vi "AlliGator Enter User-defined Phasor Dialog.vi"(8 "Error In":errorcluster, 9 "Phasor Frequency":dbl[unit], 11 "Phasor Plot Name":string) -> (0 "Error Out":errorcluster, 1 "Cancelled?":bool, 3 "New Phasor (g, s)":T4, 4 "Message":string)   [LabVIEW 2021, in "AlliGator Phasor Graph.lvlib"]
doc: "User-entered phasor dialog."
uses:
  AlliGator Phasor Graph.lvlib
  Phasor/Phasor (g, s).ctl
  Phasor/Phasor (m, phi).ctl
  Phasor/Phasor.lvlib
panel:
  in  "Prefactor Type":enum32{"Exp. Amplitude", "Intensity Fraction"}(radio)
  in  "Cancel":bool
  in  "OK":bool
  in  "Double-Exponential":T1
  in  "Single-Lifetime":dbl[unit]
  out "User Message":string
  in  "Type of Phasor Definition":T2(radio)
  in  "Phasor (m, phi)":T3
  in  "Phasor (g, s)":T4
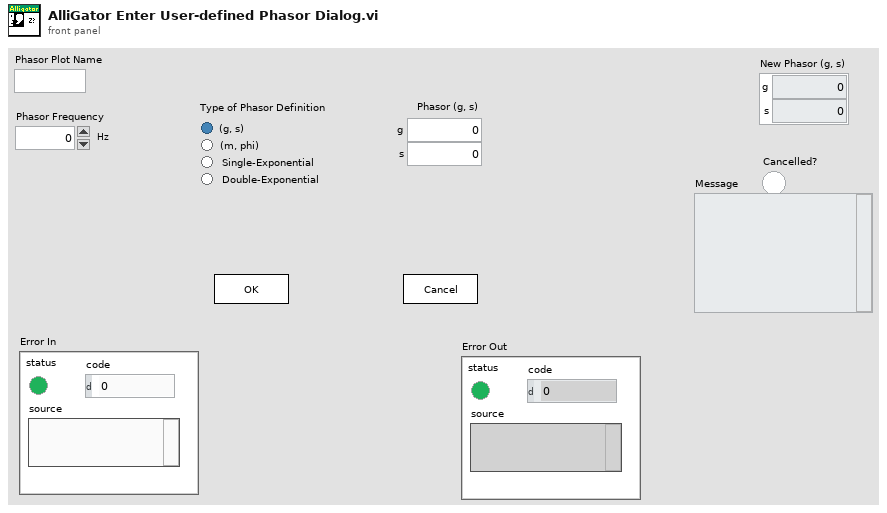
[diagram p1: front panel]
types:
  T1 = cluster{"Lifetime 1":dbl[unit], "Prefactor 1":dbl, "Lifetime 2":dbl[unit], "Prefactor 2":dbl}
  T2 = enum32{"(g, s)", "(m, phi)", "Single-Exponential", "Double-Exponential"}
  T3 = typedef "Phasor.lvlib/Phasor (m, phi).ctl" = cluster{"m":dbl, "phi":dbl}
  T4 = typedef "Phasor.lvlib/Phasor (g, s).ctl" = cluster{"g":dbl, "s":dbl}
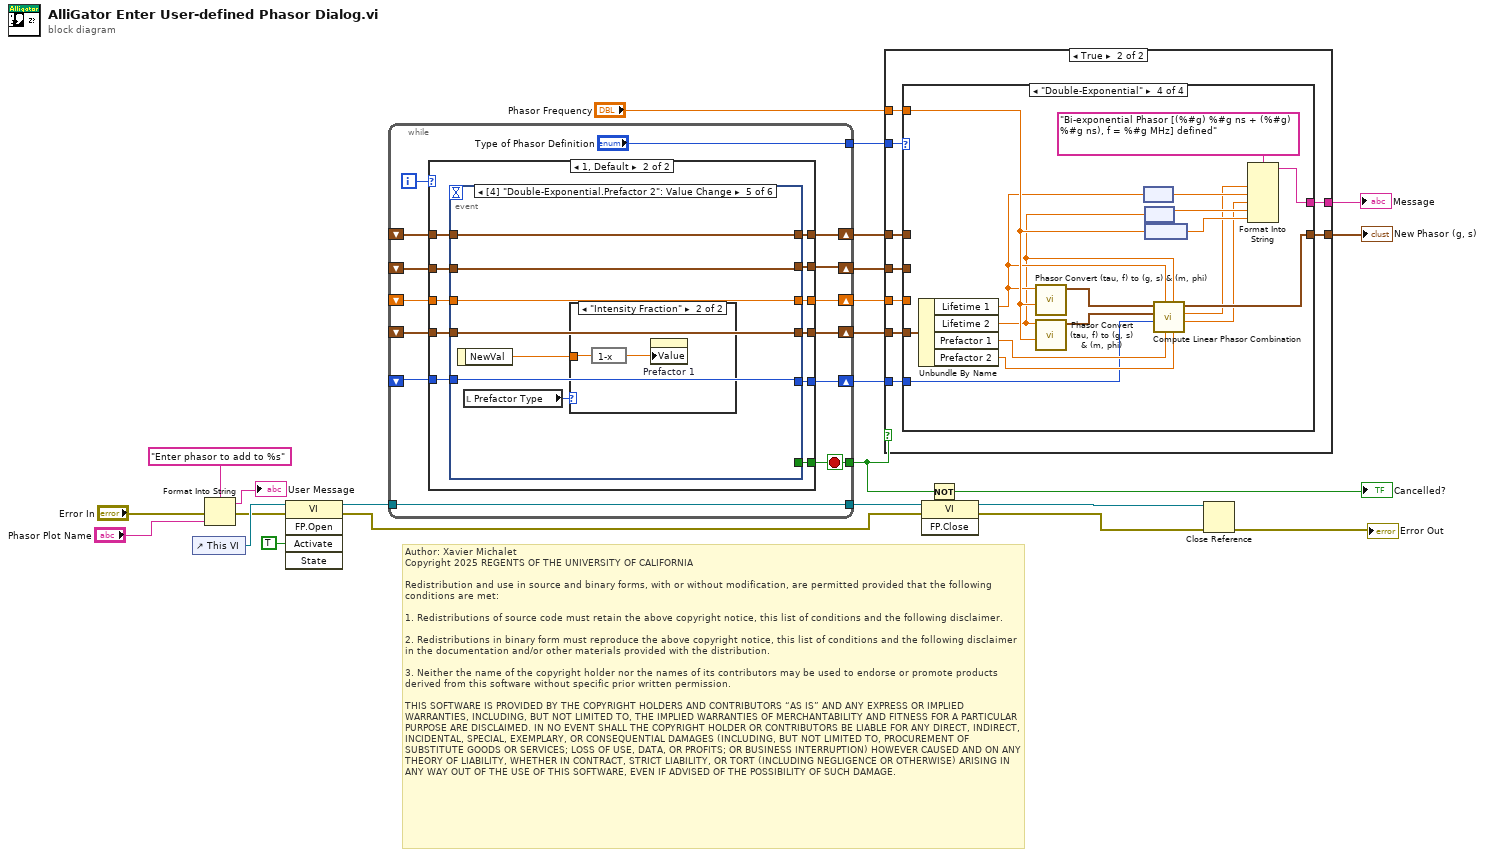
[diagram p0: block diagram]
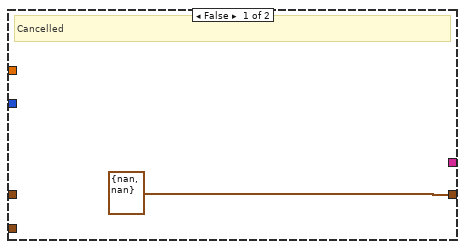
[diagram p2: hidden frame]
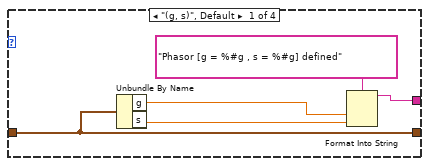
[diagram p3: hidden frame]
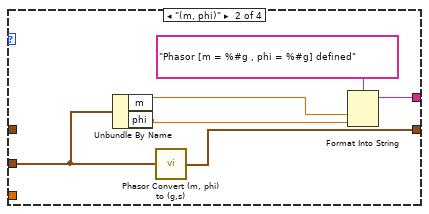
[diagram p4: hidden frame]
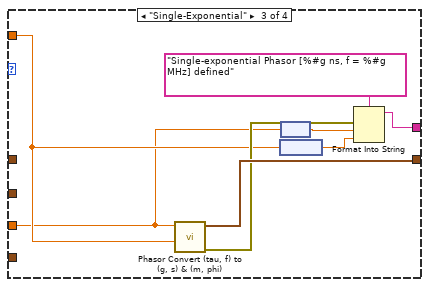
[diagram p5: hidden frame]
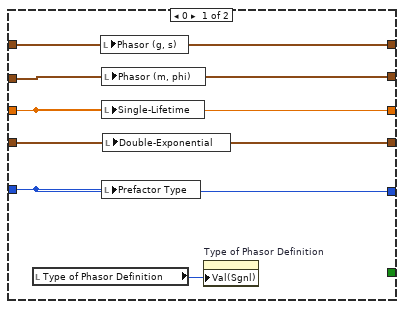
[diagram p6: hidden frame]
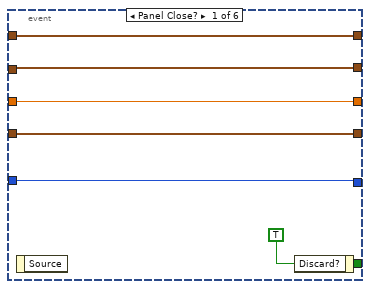
[diagram p7: hidden frame]
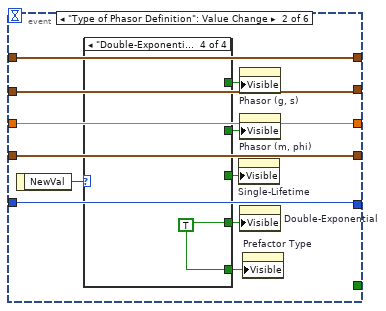
[diagram p8: hidden frame]
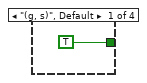
[diagram p9: hidden frame]
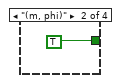
[diagram p10: hidden frame]
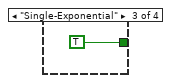
[diagram p11: hidden frame]
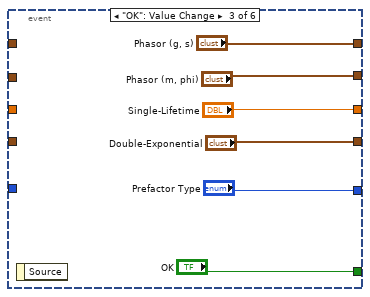
[diagram p12: hidden frame]
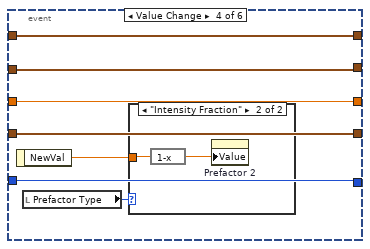
[diagram p13: hidden frame]
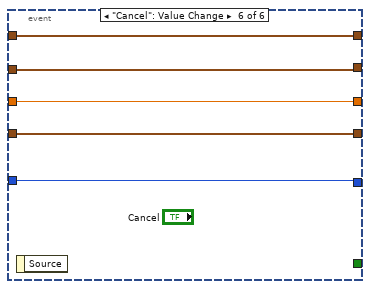
[diagram p16: hidden frame]
diagram:
  # "Author: Xavier Michalet\nCopyright 2025 REGENTS OF THE UNIVERSITY OF CALIFORNIA\n\nRedistribution and use in source and binary forms, with or without modification, are permitted provided that the following conditions are met:\n\n1. Redistributions of source code must retain the above copyright notice, this list of conditions and the following disclaimer.\n\n2. Redistributions in binary form must reproduce the above copyright notice, this list of conditions and the following disclaimer in the documentation and/or other materials provided with the distribution.\n\n3. Neither the name of the copyright holder nor the names of its contributors may be used to endorse or promote products derived from this software without specific prior written permission.\n\nTHIS SOFTWARE IS PROVIDED BY THE COPYRIGHT HOLDERS AND CONTRIBUTORS “AS IS” AND ANY EXPRESS OR IMPLIED WARRANTIES, INCLUDING, BUT NOT LIMITED TO, THE IMPLIED WARRANTIES OF MERCHANTABILITY AND FITNESS FOR A PARTICULAR PURPOSE ARE DISCLAIMED. IN NO EVENT SHALL THE COPYRIGHT HOLDER OR CONTRIBUTORS BE LIABLE FOR ANY DIRECT, INDIRECT, INCIDENTAL, SPECIAL, EXEMPLARY, OR CONSEQUENTIAL DAMAGES (INCLUDING, BUT NOT LIMITED TO, PROCUREMENT OF SUBSTITUTE GOODS OR SERVICES; LOSS OF USE, DATA, OR PROFITS; OR BUSINESS INTERRUPTION) HOWEVER CAUSED AND ON ANY THEORY OF LIABILITY, WHETHER IN CONTRACT, STRICT LIABILITY, OR TORT (INCLUDING NEGLIGENCE OR OTHERWISE) ARISING IN ANY WAY OUT OF THE USE OF THIS SOFTWARE, EVEN IF ADVISED OF THE POSSIBILITY OF SUCH DAMAGE."
  n1 = control-ref of="This VI"() -> (w24:refnum<vi>)
  n2 = Format Into String(format string="Enter phasor to add to %s", error in="Error In", "Phasor Plot Name") -> (resulting string=→"User Message":string, error out=w13:errorcluster)  [unwired: 1 in]
  n3 = invoke class="VI" method="FP.Open"(reference=w24, error in=w13, "Activate"=TRUE ("Activate?")) -> (reference out=w22:refnum<vi>, error out=w18:errorcluster)  [unwired: 2 in, 3 out]
  n4 = while {
    shift-right: [w33] -> w8
    shift-left: _ -> [w37]
    shift-right: [w32] -> w6
    shift-left: _ -> [w36]
    shift-right: [w31] -> w4
    shift-left: _ -> [w35]
    shift-right: [w30] -> w3
    shift-left: _ -> [w34]
    tunnel: ["Type of Phasor Definition"] -> w14
    tunnel: [w28] -> w15
    tunnel: w22 -> [w27]
    tunnel: [w27] -> w21
    shift-right: [w25] -> w1
    shift-left: _ -> [w26]
    i -> [w38]
    stop <- w28 stop-if-true
    n5 = case shown="1, Default" w38 {
      tunnel: [_ w55] -> w28
      tunnel: w37 -> [w44 w54]
      tunnel: w36 -> [w43 w52]
      tunnel: w35 -> [w42 w50]
      tunnel: w34 -> [w41 w48]
      tunnel: [w44 w53] -> w33
      tunnel: [w43 w51] -> w32
      tunnel: [w42 w49] -> w31
      tunnel: [w41 w47] -> w30
      tunnel: w26 -> [w39 w45]
      tunnel: [w39 w46] -> w25
      frame 0 {
        n6 = local read "Type of Phasor Definition"() -> (w40:T2)
        n7 = local write "Phasor (g, s)"(w44) -> ()
        n8 = local write "Phasor (m, phi)"(w43) -> ()
        n9 = local write "Single-Lifetime"(w42) -> ()
        n10 = local write "Prefactor Type"(w39) -> ()
        n11 = local write "Double-Exponential"(w41) -> ()
        n12 = property on="Type of Phasor Definition" class="RadioBtnsControl (strict)"("Val(Sgnl)"=w40) -> ()  [unwired: 2 in, 2 out]
      }
      frame 1, Default {
        n13 = event shown="[4] \"Double-Exponential.Prefactor 2\": Value Change" {
          selector: _ -> [_ _ _ _ _ _]
          dyn-events: _ -> [_ _ _ _ _ _]
          timeout: _ -> [_ _ _ _ _ _]
          tunnel: [w61 _ "OK" _ _ _] -> w55
          tunnel: w54 -> [w60 w67 _ w89 w98 w105]
          tunnel: [w60 w67 "Phasor (g, s)" w89 w98 w105] -> w53
          tunnel: w52 -> [w59 w66 _ w88 w97 w104]
          tunnel: [w59 w66 "Phasor (m, phi)" w88 w97 w104] -> w51
          tunnel: w50 -> [w58 w65 _ w87 w96 w103]
          tunnel: [w58 w65 "Single-Lifetime" w87 w96 w103] -> w49
          tunnel: w48 -> [w57 w64 _ w86 w95 w102]
          tunnel: [w57 w64 "Double-Exponential" w86 w95 w102] -> w47
          tunnel: [w56 w63 "Prefactor Type" w85 w94 w101] -> w46
          tunnel: w45 -> [w56 w63 _ w85 w94 w101]
          event Panel Close? {
            w61 = TRUE ("Discard?")
            n14 = event-data() -> ()  [unwired: 1 in, 1 out]
            n15 = event-data("Discard?"=w61) -> ()  [unwired: 1 in, 1 out]
          }
          event "Type of Phasor Definition": Value Change {
            n16 = event-data() -> ("NewVal"=w72:T2)  [unwired: 1 in]
            n17 = case shown="\"Double-Exponential\"" w72 {
              tunnel: [TRUE ("Visible") _ _ _] -> w71
              tunnel: [_ TRUE ("Visible") _ _] -> w70
              tunnel: [_ _ TRUE ("Visible") _] -> w69
              tunnel: [_ _ _ w76] -> w68
              tunnel: [_ _ _ w76] -> w62
              frame "(g, s)", Default {
              }
              frame "(m, phi)" {
              }
              frame "Single-Exponential" {
              }
              frame "Double-Exponential" {
                w76 = TRUE ("Visible")
              }
            }
            n18 = property on="Single-Lifetime" class="DigNum (strict)"("Visible"=w69) -> ()  [unwired: 2 in, 2 out]
            n19 = property on="Phasor (g, s)" class="Clust (strict)"("Visible"=w71) -> ()  [unwired: 2 in, 2 out]
            n20 = property on="Phasor (m, phi)" class="Clust (strict)"("Visible"=w70) -> ()  [unwired: 2 in, 2 out]
            n21 = property on="Double-Exponential" class="Clust (strict)"("Visible"=w68) -> ()  [unwired: 2 in, 2 out]
            n22 = property on="Prefactor Type" class="RadioBtnsControl (strict)"("Visible"=w62) -> ()  [unwired: 2 in, 2 out]
          }
          event "OK": Value Change {
            n23 = event-data() -> ()  [unwired: 1 in, 1 out]
          }
          event "Double-Exponential.Prefactor 1": Value Change {
            n24 = event-data() -> ("NewVal"=w83:dbl)  [unwired: 1 in]
            n25 = local read "Prefactor Type"() -> (w84:enum32{"Exp. Amplitude", "Intensity Fraction"})
            n26 = case shown="\"Intensity Fraction\"" w84 {
              tunnel: w83 -> [_ w91]
              frame "Exp. Amplitude", Default {
              }
              frame "Intensity Fraction" {
                n27 = expression code="1-x"(w91) -> (w90:dbl)
                n28 = property on="Prefactor 2" class="DigNum (strict)"("Value"=w90) -> ()  [unwired: 2 in, 2 out]
              }
            }
          }
          event "Double-Exponential.Prefactor 2": Value Change {
            n29 = event-data() -> ("NewVal"=w92:dbl)  [unwired: 1 in]
            n30 = local read "Prefactor Type"() -> (w93:enum32{"Exp. Amplitude", "Intensity Fraction"})
            n31 = case shown="\"Intensity Fraction\"" w93 {
              tunnel: w92 -> [_ w100]
              frame "Exp. Amplitude", Default {
              }
              frame "Intensity Fraction" {
                n32 = expression code="1-x"(w100) -> (w99:dbl)
                n33 = property on="Prefactor 1" class="DigNum (strict)"("Value"=w99) -> ()  [unwired: 2 in, 2 out]
              }
            }
          }
          event "Cancel": Value Change {
            n34 = event-data() -> ()  [unwired: 1 in, 1 out]
          }
        }
      }
    }
  }
  n35 = case shown="True" w15 {
    tunnel: w14 -> [_ w115]
    tunnel: w8 -> [_ w114]
    tunnel: [T4 {"g"=nan, "s"=nan} ("Phasor (g, s)") w113] -> w7
    tunnel: w6 -> [_ w112]
    tunnel: "Phasor Frequency" -> [_ w110]
    tunnel: w4 -> [_ w111]
    tunnel: w3 -> [_ w109]
    tunnel: [_ w108] -> w2
    tunnel: w1 -> [_ w107]
    frame False {
      # "Cancelled"
    }
    frame True {
      n36 = case shown="\"Double-Exponential\"" w115 {
        tunnel: w114 -> [w117 _ _ _]
        tunnel: [w117 w126 w134 w148] -> w113
        tunnel: w112 -> [_ w124 _ _]
        tunnel: w111 -> [_ _ w128 _]
        tunnel: w110 -> [_ _ w130 w142]
        tunnel: w109 -> [_ _ _ w151]
        tunnel: [w118 w125 w133 w147] -> w108
        tunnel: w107 -> [_ _ _ w137]
        frame "(g, s)", Default {
          n37 = Unbundle By Name(w117) -> ("g"=w120:dbl, "s"=w116:dbl)
          n38 = Format Into String(format string="Phasor [g = %#g , s = %#g] defined", w120, w116) -> (resulting string=w118:string)  [unwired: 2 in, 1 out]
        }
        frame "(m, phi)" {
          n39 = Unbundle By Name(w124) -> ("m"=w123:dbl, "phi"=w122:dbl)
          n40 = call "Phasor Convert (m, phi) to (g,s).vi"("Phasor (m, phi)"=w124) -> ("Phasor (g, s)"=w126:T4)  [unwired: 8 in]
          n41 = Format Into String(format string="Phasor [m = %#g , phi = %#g] defined", w123, w122) -> (resulting string=w125:string)  [unwired: 2 in, 1 out]
        }
        frame "Single-Exponential" {
          n42 = call "Phasor Convert (tau, f) to (g, s) & (m, phi).vi"("Phasor Frequency"=w130, "Phase Lifetime"=w128) -> ("Error Out"=w132:errorcluster, "Phasor (g, s)"=w134:T4)  [unwired: 7 in, 1 out]
          n43 = node(w130) -> (w131:dbl)
          n44 = node(w128) -> (w129:dbl)
          n45 = Format Into String(format string="Single-exponential Phasor [%#g ns, f = %#g MHz] defined", error in=w132, w129, w131) -> (resulting string=w133:string)  [unwired: 1 in, 1 out]
        }
        frame "Double-Exponential" {
          n46 = Unbundle By Name(w151) -> ("Lifetime 1"=w139:dbl[unit], "Lifetime 2"=w138:dbl[unit], "Prefactor 1"=w141:dbl, "Prefactor 2"=w140:dbl)
          n47 = call "Phasor Convert (tau, f) to (g, s) & (m, phi).vi"("Phasor Frequency"=w142, "Phase Lifetime"=w139) -> ("Phasor (g, s)"=w150:T4)  [unwired: 7 in, 2 out]
          n48 = call "Phasor Convert (tau, f) to (g, s) & (m, phi).vi"("Phasor Frequency"=w142, "Phase Lifetime"=w138) -> ("Phasor (g, s)"=w149:T4)  [unwired: 7 in, 2 out]
          n49 = node(w139) -> (w145:dbl)
          n50 = node(w138) -> (w144:dbl)
          n51 = node(w142) -> (w143:dbl)
          n52 = call "Compute Linear Phasor Combination.vi"("Prefactor 2"=w140, "Lifetime 2"=w138, "Prefactor 1"=w141, "Lifetime 1"=w139, "Prefactor Type"=w137, "Phasor 2"=w149, "Phasor 1"=w150) -> ("f2"=w135:dbl, "f1"=w136:dbl, "Phasor (g, s) out"=w148:T4)  [unwired: 2 in]
          n53 = Format Into String(format string="Bi-exponential Phasor [(%#g) %#g ns + (%#g) %#g ns), f = %#g MHz] defined", w136, w145, w135, w144, w143) -> (resulting string=w147:string)  [unwired: 2 in, 1 out]
        }
      }
    }
  }
  "New Phasor (g, s)" <- w7
  "Message" <- w2
  n54 = invoke class="VI" method="FP.Close"(reference=w21, error in=w18) -> (reference out=w20:refnum<vi>, error out=w19:errorcluster)  [unwired: 1 in, 1 out]
  n55 = Not(x=w15) -> (.not. x?=→"Cancelled?":bool)
  n56 = Close Reference(reference=w20, error in (no error)=w19) -> (error out=→"Error Out":errorcluster)
